vi "AnimatorConfig.vi"(0 "State In":T4 caption="State", 11 "error in (no error)":errorcluster) -> (4 "State Out":T4 caption="State", 8 "Cancel?":bool, 15 "error out":errorcluster)   [LabVIEW 2013, in "AnimatorXControl.xctl"]
uses:
  AnimatorXControl.xctl
  AnimatorState.ctl
  <vilib>/picture/picture.llb/imagedata.ctl
  AnimatorSettings.ctl
  DefaultImageData.vi
  Instance           1 22Saved   AnimatorConfig .vi
panel:
  in  "Cluster":T2
  out "ImageTemp":T3
  out "PathTemp":path
  in  "Reverse":bool
  in  "Frame rate (fps)":dbl
  in  "Animation Settings":enum32{"Automatic", "UseValue"}(radio)
  out "Animation Preview":picture
  in  "Help":bool
  in  "Cancel":bool
  in  "OK":bool
  in  "Down":bool
  in  "Up":bool
  in  "RemoveAll":bool
  in  "Remove":bool
  in  "Add":bool
  in  "Animation Images":i32(listbox)
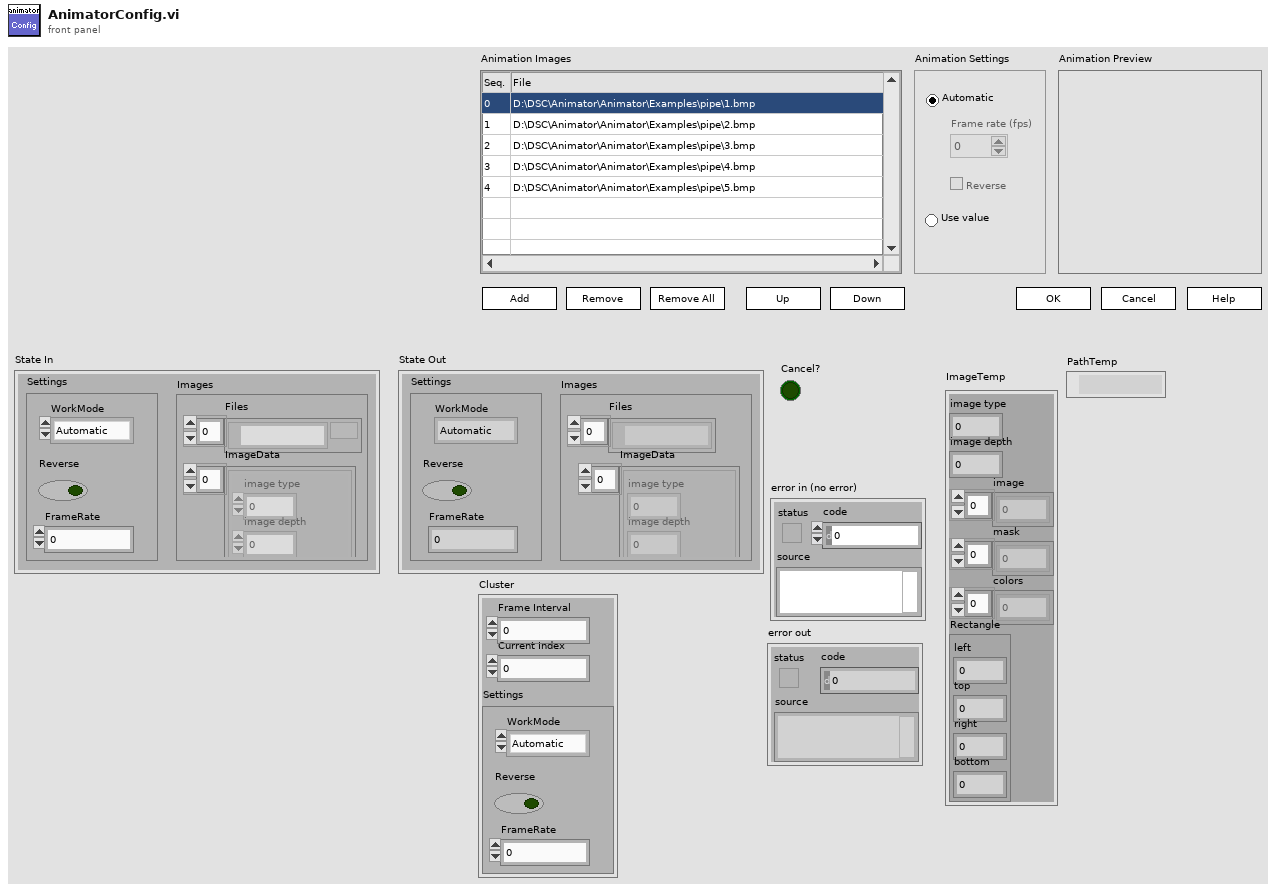
[diagram p1: front panel]
types:
  T1 = typedef "AnimatorXControl.xctl/AnimatorSettings.ctl" = cluster{"Reverse":bool, "FrameRate":dbl, "WorkMode":enum16{"Automatic", "UseValue"}}
  T2 = cluster{"Frame Interval":dbl, "Current Index":u32, "Settings":T1}
  T3 = typedef "imagedata.ctl" = cluster{"image type":i32, "image depth":i32, "image":u8[], "mask":u8[], "colors":u32[], "Rectangle":cluster{"left":i16, "top":i16, "right":i16, "bottom":i16}}
  T4 = typedef "AnimatorXControl.xctl/AnimatorState.ctl" = cluster{"Images":cluster{"Files":path[], "ImageData":T3[]}, "Settings":T1}
  T5 = enum16{"Add", "Remove", "RemoveAll", "MoveUp", "MoveDown"}
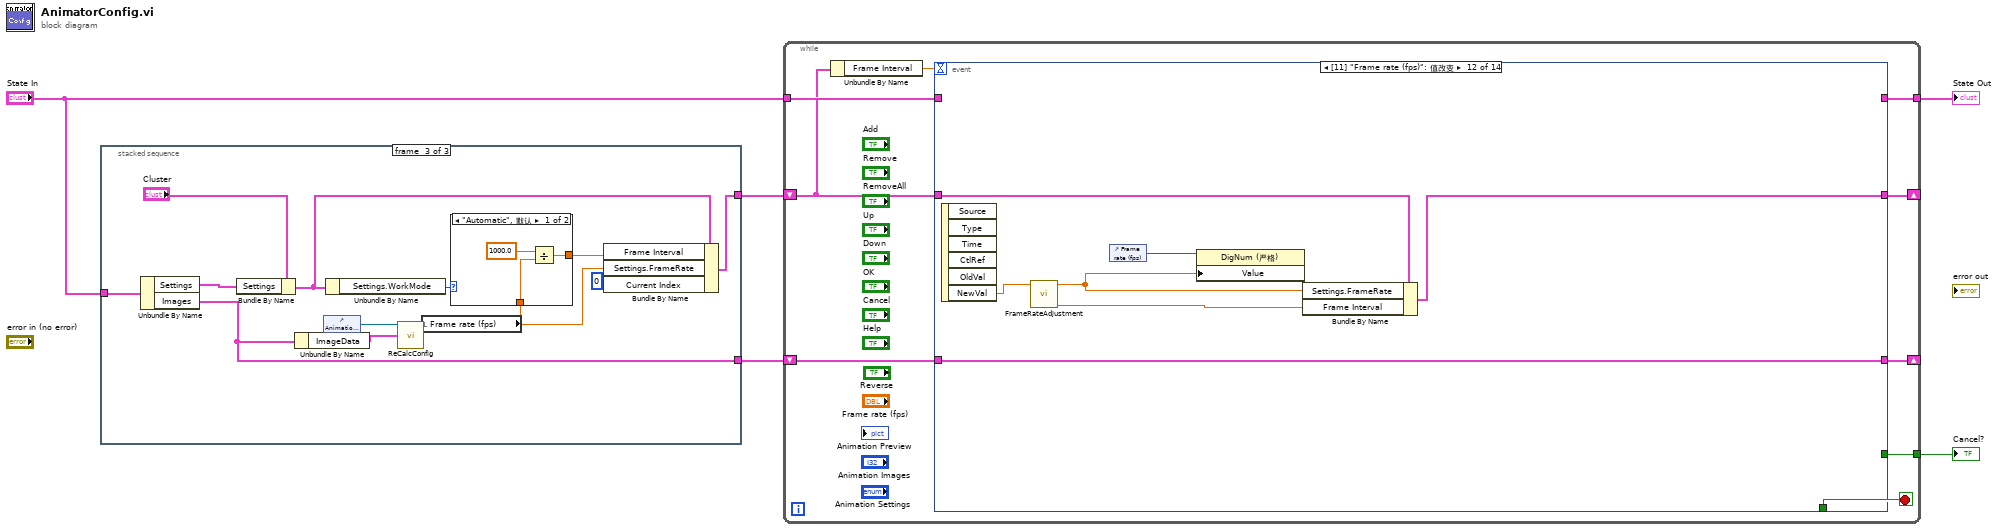
[diagram p0: block diagram]
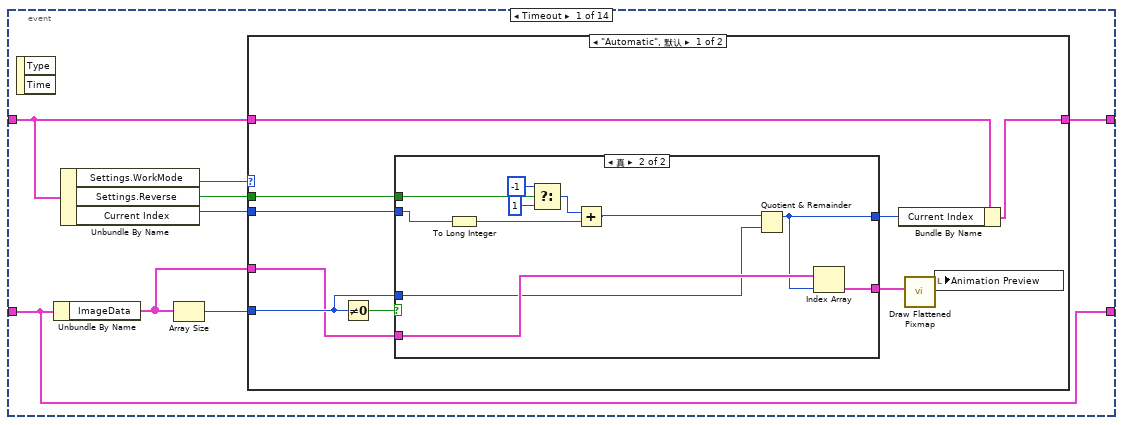
[diagram p2: hidden frame]
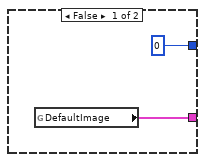
[diagram p3: hidden frame]
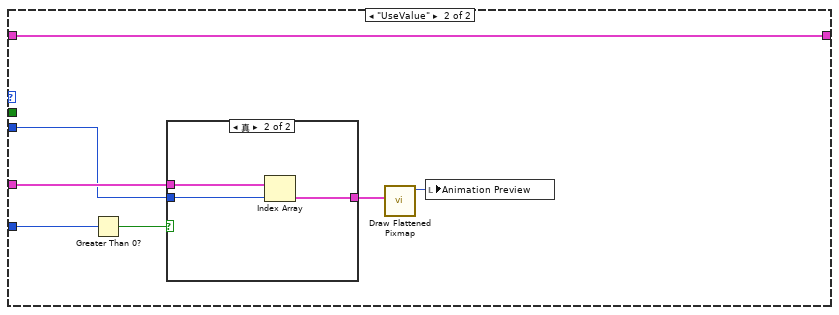
[diagram p4: hidden frame]
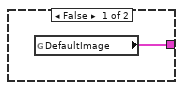
[diagram p5: hidden frame]
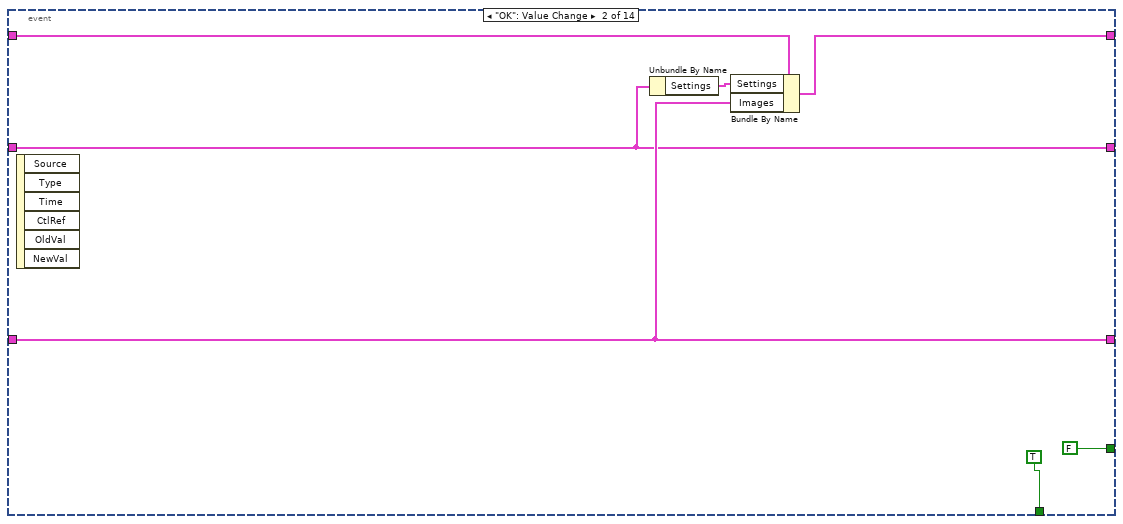
[diagram p6: hidden frame]
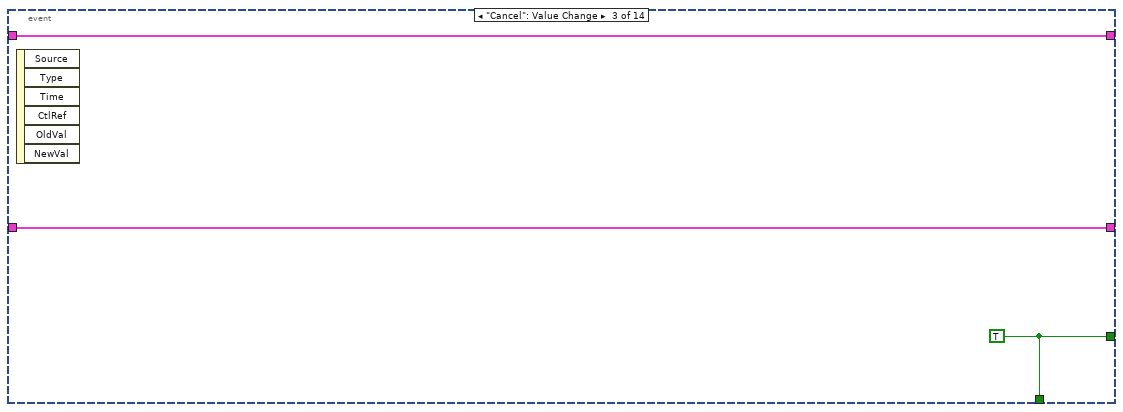
[diagram p7: hidden frame]
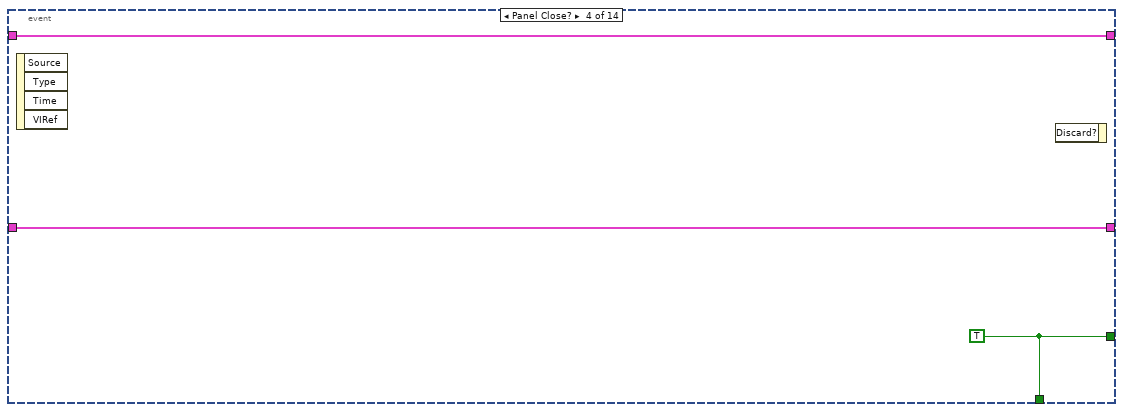
[diagram p8: hidden frame]
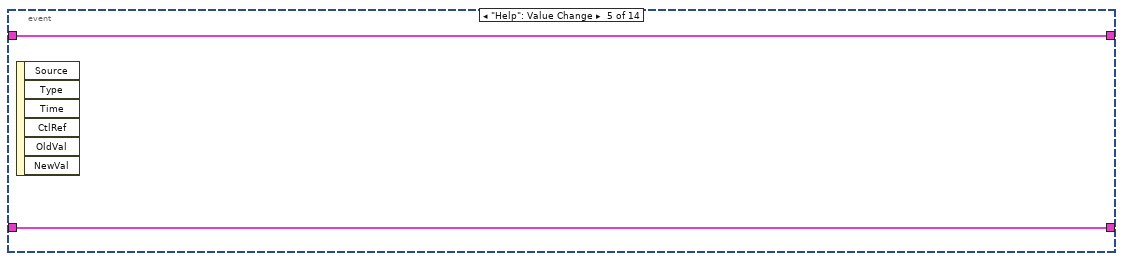
[diagram p9: hidden frame]
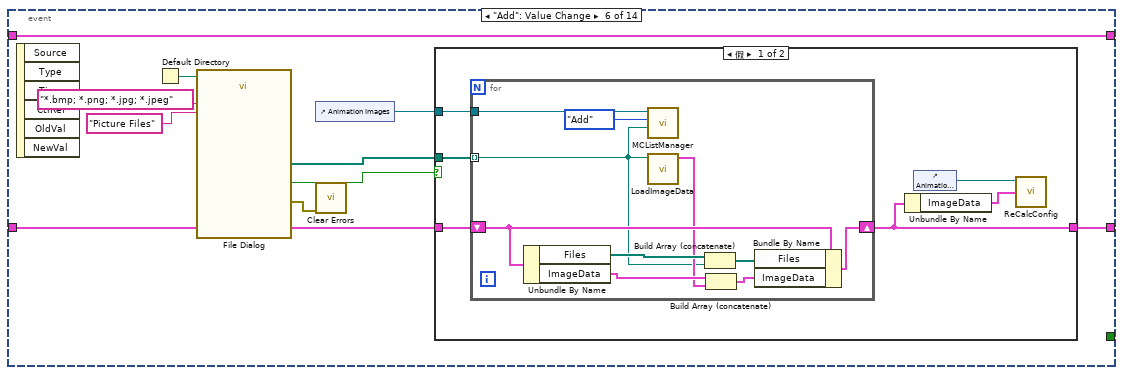
[diagram p10: hidden frame]
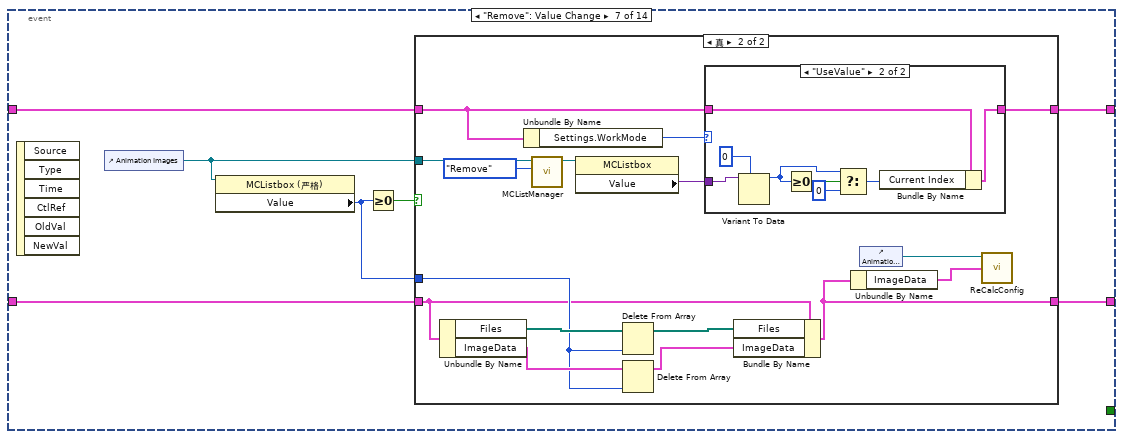
[diagram p12: hidden frame]
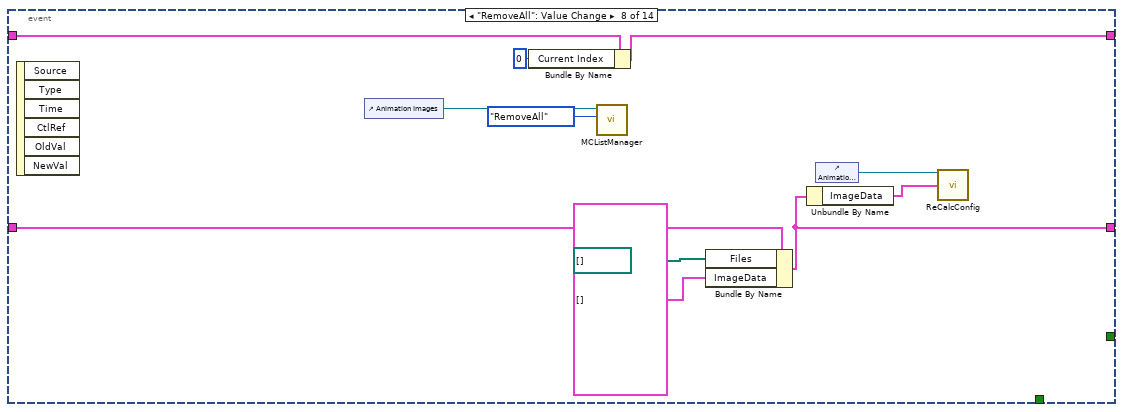
[diagram p15: hidden frame]
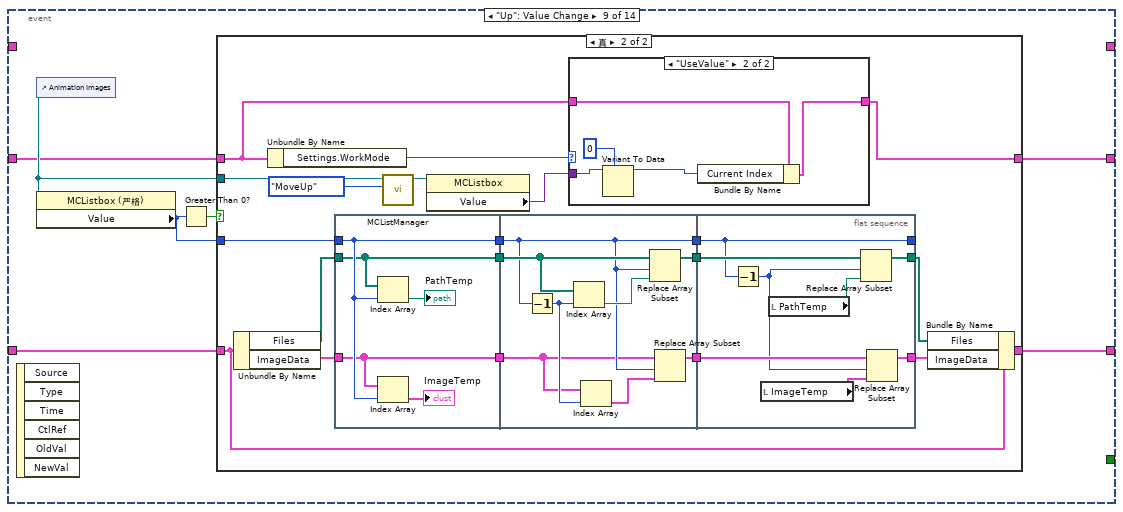
[diagram p16: hidden frame]
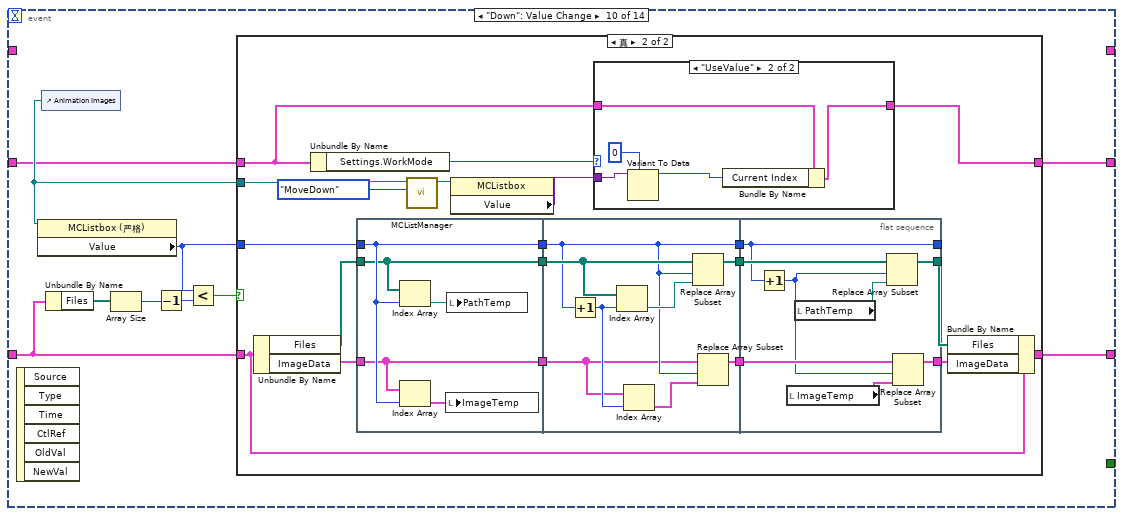
[diagram p19: hidden frame]
diagram:
  n1 = stacked-sequence {
    tunnel: "State In" -> [w22 w31 w46]
    tunnel: [_ _ w44] -> w5
    tunnel: [_ _ w43] -> w4
    frame #0 {
      n2 = Unbundle By Name(w22) -> ("Settings.WorkMode"=w8:enum16{"Automatic", "UseValue"}, "Settings.Reverse"=w17:bool, "Settings.FrameRate"=w11:dbl)
      n3 = case shown="\"UseValue\"" w8 {
        tunnel: [0 ("f") 2 ("t")] -> w7
        tunnel: [enum32{"Automatic", "UseValue"}."Automatic" ("Animation Settings") enum32{"Automatic", "UseValue"}."UseValue" ("Animation Settings")] -> w6
        frame "Automatic", Default {
        }
        frame "UseValue" {
        }
      }
      n4 = local write "Animation Settings"(w6) -> ()
      n5 = control-ref of="Frame rate (fps)"() -> (w21:refnum<vi>)
      n6 = control-ref of="Reverse"() -> (w20:refnum<vi>)
      n7 = Greater?(x=w11, y=25.0) -> (0:w14:bool)
      n8 = Less?(x=w11, y=0.1) -> (x < y?=w13:bool)
      n9 = Not Or(1:w13, 2:w14) -> (0:w10:bool)
      n10 = property class="DigNum (严格)"(reference=w21, "Disabled"=w7) -> (reference out=w19:refnum<vi>)  [unwired: 1 in, 1 out]
      n11 = Select(t=w11, s=w10, f=1.0) -> (s? t:f=w9:dbl)
      n12 = property class="Bool (严格)"(reference=w20, "Disabled"=w7) -> (reference out=w18:refnum<vi>)  [unwired: 1 in, 1 out]
      n13 = property class="DigNum (严格)"(reference=w19, "Value"=w9) -> ()  [unwired: 1 in, 2 out]
      n14 = property class="Bool (严格)"(reference=w18, "Value"=w17) -> ()  [unwired: 1 in, 2 out]
    }
    frame #1 {
      n15 = Unbundle By Name(w31) -> ("Images.Files"=w30:path[])
      n16 = control-ref of="Animation Images"() -> (w29:refnum<vi>)
      n17 = call "MCListManager.vi"("Command"=T5."RemoveAll", "MCListbox Refnum"=w29) -> ("MCListbox Refnum out"=w27:refnum<vi>)  [unwired: 8 in, 1 out]
      n18 = for {
        tunnel: w30 -> [w33] mode=indexing
        tunnel: w27 -> [w34]
        n19 = call "MCListManager.vi"("Path"=w33, "Command"=T5."Add", "MCListbox Refnum"=w34) -> ()  [unwired: 7 in, 2 out]
      }
    }
    frame #2 {
      n20 = Unbundle By Name(w46) -> ("Settings"=w45:T1, "Images"=w43:cluster{"Files":path[], "ImageData":T3[]})
      n21 = Bundle By Name(cluster="Cluster", "Settings"=w45) -> (w42:T2)
      n22 = Unbundle By Name(w43) -> ("ImageData"=w39:T3[])
      n23 = control-ref of="Animation Preview"() -> (w38:refnum<vi>)
      n24 = Unbundle By Name(w42) -> ("Settings.WorkMode"=w37:enum16{"Automatic", "UseValue"})
      n25 = call "ReCalcConfig.vi"("Pict Refnum"=w38, "Image Array"=w39) -> ()  [unwired: 13 in, 1 out]
      n26 = local read "Frame rate (fps)"() -> (w35:dbl)
      n27 = case shown="\"Automatic\", 默认" w37 {
        tunnel: [w49 40.0] -> w36
        tunnel: w35 -> [w48 _]
        frame "Automatic", Default {
          n28 = Divide(x=1000.0, y=w48) -> (x/y=w49:dbl)
        }
        frame "UseValue" {
        }
      }
      n29 = Bundle By Name(cluster=w42, "Frame Interval"=w36, "Settings.FrameRate"=w35, "Current Index"=u32 0) -> (w44:T2)
    }
  }
  n30 = while {
    shift-right: [w57] -> _
    shift-left: w4 -> [w59]
    shift-right: [w58] -> _
    shift-left: w5 -> [w52]
    tunnel: [w55] -> w3
    tunnel: "State In" -> [w54]
    tunnel: [w53] -> w1
    stop <- w56 stop-if-true
    n31 = Unbundle By Name(w52) -> ("Frame Interval"=w51:dbl)
    n32 = event shown="[11] \"Frame rate (fps)\": 值改变" {
      selector: _ -> [_ _ _ _ _ _ _ _ _ _ _ _ _ _]
      dyn-events: _ -> [_ _ _ _ _ _ _ _ _ _ _ _ _ _]
      timeout: w51 -> [_ _ _ _ _ _ _ _ _ _ _ _ _ _]
      tunnel: w52 -> [w64 w103 w111 w114 w116 w124 w145 w184 w190 w246 w307 w334 w339 w342]
      tunnel: w59 -> [w60 w105 w110 w113 w115 w122 w149 w188 w192 w250 w305 w331 w337 w344]
      tunnel: [w63 w103 w111 w114 w116 w124 w144 w182 w189 w245 w306 w333 w338 w341] -> w58
      tunnel: [w60 w105 w110 w113 w115 w121 w148 w185 w191 w251 w305 w331 w337 w344] -> w57
      tunnel: [_ TRUE w109 w112 _ _ _ _ _ _ _ _ _ _] -> w56
      tunnel: [_ FALSE w109 w112 _ _ _ _ _ _ _ _ _ _] -> w55
      tunnel: w54 -> [_ w104 _ _ _ _ _ _ _ _ _ _ _ _]
      tunnel: [_ w106 _ _ _ _ _ _ _ _ _ _ _ _] -> w53
      event Timeout {
        n33 = event-data() -> ()  [unwired: 1 in, 2 out]
        n34 = Unbundle By Name(w60) -> ("ImageData"=w61:T3[])
        n35 = Unbundle By Name(w64) -> ("Settings.WorkMode"=w67:enum16{"Automatic", "UseValue"}, "Settings.Reverse"=w66:bool, "Current Index"=w62:u32)
        n36 = Array Size(array=w61) -> (size(s)=w65:i32)
        n37 = case shown="\"Automatic\", 默认" w67 {
          tunnel: w66 -> [w77 _]
          tunnel: w65 -> [w76 w93]
          tunnel: w61 -> [w75 w92]
          tunnel: w64 -> [w74 w97]
          tunnel: [w73 w97] -> w63
          tunnel: w62 -> [w72 w91]
          frame "Automatic", Default {
            n38 = Not Equal To 0?(x=w76) -> (x != 0?=w71:bool)
            n39 = case shown="真" w71 {
              tunnel: w77 -> [_ w87]
              tunnel: w76 -> [_ w85]
              tunnel: w75 -> [_ w86]
              tunnel: [w79 w84] -> w70
              tunnel: [0 w83] -> w68
              tunnel: w72 -> [_ w82]
              frame False {
                n40 = global read "DefaultImageData.vi" "DefaultImage"() -> (w79:T3)
              }
              frame True {
                n41 = To Long Integer(number=w82) -> (32bit integer=w81:i32)
                n42 = Select(t=-1, s=w87, f=1) -> (s? t:f=w90:i32)
                n43 = Add(x=w90, y=w81) -> (x+y=w80:i32)
                n44 = Quotient & Remainder(x=w80, y=w85) -> (x-y*floor(x/y)=w83:i32)  [unwired: 1 out]
                n45 = Index Array(array=w86, index=w83) -> (element=w84:T3)
              }
            }
            n46 = Bundle By Name(cluster=w74, "Current Index"=w68) -> (w73:T2)
            n47 = call <vilib>:"Draw Flattened Pixmap.vi"("image data"=w70) -> ("new picture"=w69:picture)  [unwired: 8 in]
            n48 = local write "Animation Preview"(w69) -> ()
          }
          frame "UseValue" {
            n49 = Greater Than 0?(x=w93) -> (x > 0?=w94:bool)
            n50 = case shown="真" w94 {
              tunnel: w92 -> [_ w101]
              tunnel: w91 -> [_ w100]
              tunnel: [w98 w99] -> w96
              frame False {
                n51 = global read "DefaultImageData.vi" "DefaultImage"() -> (w98:T3)
              }
              frame True {
                n52 = Index Array(array=w101, index=w100) -> (element=w99:T3)
              }
            }
            n53 = call <vilib>:"Draw Flattened Pixmap.vi"("image data"=w96) -> ("new picture"=w95:picture)  [unwired: 8 in]
            n54 = local write "Animation Preview"(w95) -> ()
          }
        }
      }
      event "OK": Value Change {
        n55 = event-data() -> ()  [unwired: 1 in, 6 out]
        n56 = Unbundle By Name(w103) -> ("Settings"=w107:T1)
        n57 = Bundle By Name(cluster=w104, "Settings"=w107, "Images"=w105) -> (w106:T4)
      }
      event "Cancel": Value Change {
        w109 = TRUE
        n58 = event-data() -> ()  [unwired: 1 in, 6 out]
      }
      event Panel Close? {
        w112 = TRUE
        n59 = event-data() -> ()  [unwired: 1 in, 4 out]
        n60 = event-data() -> ()  [unwired: 2 in, 1 out]
      }
      event "Help": Value Change {
        n61 = event-data() -> ()  [unwired: 1 in, 6 out]
      }
      event "Add": Value Change {
        n62 = event-data() -> ()  [unwired: 1 in, 6 out]
        n63 = Default Directory() -> (w119:path)
        n64 = call "File Dialog"("start path"=w119, "pattern (all files)"="*.bmp; *.png; *.jpg; *.jpeg", "pattern label"="Picture Files") -> ("selected paths"=w123:path[], "cancelled"=w117:bool, "error out"=w118:errorcluster)  [unwired: 9 in, 1 out]
        n65 = control-ref of="Animation Images"() -> (w120:refnum<vi>)
        n66 = call <vilib>:"Clear Errors.vi"("error in (no error)"=w118) -> ()  [unwired: 6 in, 1 out]
        n67 = case shown="假" w117 {
          tunnel: w123 -> [w132 _]
          tunnel: w122 -> [w131 w143]
          tunnel: [w127 w143] -> w121
          tunnel: w120 -> [w130 _]
          frame False {
            n68 = for {
              tunnel: w132 -> [w133] mode=indexing
              shift-right: [w136] -> w127
              shift-left: w131 -> [w140]
              tunnel: w130 -> [w135]
              n69 = Unbundle By Name(w140) -> ("Files"=w141:path[], "ImageData"=w142:T3[])
              n70 = call "MCListManager.vi"("Path"=w133, "Command"=T5."Add", "MCListbox Refnum"=w135) -> ()  [unwired: 7 in, 2 out]
              n71 = call "LoadImageData.vi"("path"=w133) -> ("image data"=w139:T3)  [unwired: 9 in, 1 out]
              n72 = Build Array (concatenate)(w141, w133) -> (w138:path[])
              n73 = Build Array (concatenate)(w142, w139) -> (w137:T3[])
              n74 = Bundle By Name(cluster=w140, "Files"=w138, "ImageData"=w137) -> (w136:cluster{"Files":path[], "ImageData":T3[]})
            }
            n75 = Unbundle By Name(w127) -> ("ImageData"=w129:T3[])
            n76 = control-ref of="Animation Preview"() -> (w128:refnum<vi>)
            n77 = call "ReCalcConfig.vi"("Pict Refnum"=w128, "Image Array"=w129) -> ()  [unwired: 13 in, 1 out]
          }
          frame True {
          }
        }
      }
      event "Remove": Value Change {
        n78 = event-data() -> ()  [unwired: 1 in, 6 out]
        n79 = control-ref of="Animation Images"() -> (w147:refnum<vi>)
        n80 = property class="MCListbox (严格)"(reference=w147) -> ("Value"=w146:i32)  [unwired: 1 in, 2 out]
        n81 = Greater Or Equal To 0?(x=w146) -> (x >= 0?=w150:bool)
        n82 = case shown="真" w150 {
          tunnel: w149 -> [w152 w163]
          tunnel: [w152 w160] -> w148
          tunnel: w147 -> [_ w167]
          tunnel: w146 -> [_ w164]
          tunnel: w145 -> [w151 w157]
          tunnel: [w151 w156] -> w144
          frame False {
          }
          frame True {
            n83 = Unbundle By Name(w163) -> ("Files"=w166:path[], "ImageData"=w165:T3[])
            n84 = Unbundle By Name(w157) -> ("Settings.WorkMode"=w158:enum16{"Automatic", "UseValue"})
            n85 = call "MCListManager.vi"("Command"=T5."Remove", "MCListbox Refnum"=w167) -> ("MCListbox Refnum out"=w159:refnum<vi>)  [unwired: 8 in, 1 out]
            n86 = property class="MCListbox"(reference=w159) -> ("Value"=w155:variant)  [unwired: 1 in, 2 out]
            n87 = Delete From Array(array=w166, index=w164) -> (array with subset deleted=w162:path[])  [unwired: 1 in, 1 out]
            n88 = Delete From Array(array=w165, index=w164) -> (array with subset deleted=w161:T3[])  [unwired: 1 in, 1 out]
            n89 = case shown="\"UseValue\"" w158 {
              tunnel: w157 -> [w169 w175]
              tunnel: [w169 w174] -> w156
              tunnel: w155 -> [_ w177]
              frame "Automatic", Default {
              }
              frame "UseValue" {
                n90 = Variant To Data(type=0, Variant=w177) -> (data=w171:i32)  [unwired: 1 in, 1 out]
                n91 = Greater Or Equal To 0?(x=w171) -> (x >= 0?=w173:bool)
                n92 = Select(t=w171, s=w173, f=0) -> (s? t:f=w172:i32)
                n93 = Bundle By Name(cluster=w175, "Current Index"=w172) -> (w174:T2)
              }
            }
            n94 = Bundle By Name(cluster=w163, "Files"=w162, "ImageData"=w161) -> (w160:cluster{"Files":path[], "ImageData":T3[]})
            n95 = Unbundle By Name(w160) -> ("ImageData"=w153:T3[])
            n96 = control-ref of="Animation Preview"() -> (w154:refnum<vi>)
            n97 = call "ReCalcConfig.vi"("Pict Refnum"=w154, "Image Array"=w153) -> ()  [unwired: 13 in, 1 out]
          }
        }
      }
      event "RemoveAll": Value Change {
        n98 = event-data() -> ()  [unwired: 1 in, 6 out]
        n99 = control-ref of="Animation Images"() -> (w187:refnum<vi>)
        n100 = Bundle By Name(cluster=w184, "Current Index"=u32 0) -> (w182:T2)
        n101 = call "MCListManager.vi"("Command"=T5."RemoveAll", "MCListbox Refnum"=w187) -> ()  [unwired: 8 in, 2 out]
        n102 = Bundle By Name(cluster=w188, "Files"=path[] [], "ImageData"=T3[] []) -> (w185:cluster{"Files":path[], "ImageData":T3[]})
        n103 = Unbundle By Name(w185) -> ("ImageData"=w178:T3[])
        n104 = control-ref of="Animation Preview"() -> (w179:refnum<vi>)
        n105 = call "ReCalcConfig.vi"("Pict Refnum"=w179, "Image Array"=w178) -> ()  [unwired: 13 in, 1 out]
      }
      event "Up": Value Change {
        n106 = event-data() -> ()  [unwired: 1 in, 6 out]
        n107 = control-ref of="Animation Images"() -> (w194:refnum<vi>)
        n108 = property class="MCListbox (严格)"(reference=w194) -> ("Value"=w193:i32)  [unwired: 1 in, 2 out]
        n109 = Greater Than 0?(x=w193) -> (x > 0?=w195:bool)
        n110 = case shown="真" w195 {
          tunnel: w194 -> [_ w216]
          tunnel: w193 -> [_ w214]
          tunnel: w192 -> [w197 w203]
          tunnel: [w197 w204] -> w191
          tunnel: w190 -> [w196 w199]
          tunnel: [w196 w198] -> w189
          frame False {
          }
          frame True {
            n111 = Unbundle By Name(w203) -> ("Files"=w208:path[], "ImageData"=w207:T3[])
            n112 = Unbundle By Name(w199) -> ("Settings.WorkMode"=w202:enum16{"Automatic", "UseValue"})
            n113 = flat-sequence {
              tunnel: [w228] -> w215
              tunnel: w214 -> [w228]
              tunnel: w208 -> [w225]
              tunnel: w207 -> [w224]
              tunnel: [w225] -> w212
              tunnel: [w224] -> w211
              tunnel: w215 -> [w233]
              tunnel: [w233] -> w213
              tunnel: w212 -> [w235]
              tunnel: w211 -> [w231]
              tunnel: [w230] -> w210
              tunnel: [w229] -> w209
              tunnel: [w242] -> _
              tunnel: w213 -> [w242]
              tunnel: w210 -> [w244]
              tunnel: w209 -> [w243]
              tunnel: [w238] -> w205
              tunnel: [w237] -> w206
              frame #0 {
                n114 = Index Array(array=w225, index=w228) -> (element=→"PathTemp":path)
                n115 = Index Array(array=w224, index=w228) -> (element=→"ImageTemp":T3)
              }
              frame #1 {
                n116 = Decrement(x=w233) -> (x-1=w236:i32)
                n117 = Index Array(array=w235, index=w236) -> (element=w234:path)
                n118 = Index Array(array=w231, index=w236) -> (element=w232:T3)
                n119 = Replace Array Subset(array=w235, new element=w234, index=w233) -> (w230:path[])
                n120 = Replace Array Subset(array=w231, new element=w232, index=w233) -> (w229:T3[])
              }
              frame #2 {
                n121 = Decrement(x=w242) -> (x-1=w241:i32)
                n122 = local read "ImageTemp"() -> (w239:T3)
                n123 = local read "PathTemp"() -> (w240:path)
                n124 = Replace Array Subset(array=w244, new element=w240, index=w241) -> (w238:path[])
                n125 = Replace Array Subset(array=w243, new element=w239, index=w241) -> (w237:T3[])
              }
            }
            n126 = call "MCListManager.vi"("Command"=T5."MoveUp", "MCListbox Refnum"=w216) -> ("MCListbox Refnum out"=w201:refnum<vi>)  [unwired: 8 in, 1 out]
            n127 = property class="MCListbox"(reference=w201) -> ("Value"=w200:variant)  [unwired: 1 in, 2 out]
            n128 = case shown="\"UseValue\"" w202 {
              tunnel: w199 -> [w218 w221]
              tunnel: [w218 w219] -> w198
              tunnel: w200 -> [_ w223]
              frame "Automatic", Default {
              }
              frame "UseValue" {
                n129 = Variant To Data(type=0, Variant=w223) -> (data=w220:i32)  [unwired: 1 in, 1 out]
                n130 = Bundle By Name(cluster=w221, "Current Index"=w220) -> (w219:T2)
              }
            }
            n131 = Bundle By Name(cluster=w203, "Files"=w205, "ImageData"=w206) -> (w204:cluster{"Files":path[], "ImageData":T3[]})
          }
        }
      }
      event "Down": Value Change {
        n132 = event-data() -> ()  [unwired: 1 in, 6 out]
        n133 = control-ref of="Animation Images"() -> (w247:refnum<vi>)
        n134 = property class="MCListbox (严格)"(reference=w247) -> ("Value"=w249:i32)  [unwired: 1 in, 2 out]
        n135 = Unbundle By Name(w250) -> ("Files"=w254:path[])
        n136 = Array Size(array=w254) -> (size(s)=w253:i32)
        n137 = Decrement(x=w253) -> (x-1=w252:i32)
        n138 = Less?(x=w249, y=w252) -> (x < y?=w248:bool)
        n139 = case shown="真" w248 {
          tunnel: w247 -> [_ w275]
          tunnel: w249 -> [_ w273]
          tunnel: w250 -> [w256 w262]
          tunnel: [w256 w263] -> w251
          tunnel: w246 -> [w255 w260]
          tunnel: [w255 w257] -> w245
          frame False {
          }
          frame True {
            n140 = Unbundle By Name(w262) -> ("Files"=w267:path[], "ImageData"=w266:T3[])
            n141 = Unbundle By Name(w260) -> ("Settings.WorkMode"=w259:enum16{"Automatic", "UseValue"})
            n142 = flat-sequence {
              tunnel: [w287] -> w274
              tunnel: w273 -> [w287]
              tunnel: w267 -> [w286]
              tunnel: w266 -> [w285]
              tunnel: [w286] -> w271
              tunnel: [w285] -> w270
              tunnel: w274 -> [w292]
              tunnel: [w292] -> w272
              tunnel: w271 -> [w294]
              tunnel: w270 -> [w290]
              tunnel: [w289] -> w269
              tunnel: [w288] -> w268
              tunnel: [w301] -> _
              tunnel: w272 -> [w301]
              tunnel: w269 -> [w303]
              tunnel: w268 -> [w302]
              tunnel: [w297] -> w264
              tunnel: [w296] -> w265
              frame #0 {
                n143 = Index Array(array=w286, index=w287) -> (element=w284:path)
                n144 = Index Array(array=w285, index=w287) -> (element=w283:T3)
                n145 = local write "ImageTemp"(w283) -> ()
                n146 = local write "PathTemp"(w284) -> ()
              }
              frame #1 {
                n147 = Increment(x=w292) -> (x+1=w295:i32)
                n148 = Index Array(array=w294, index=w295) -> (element=w293:path)
                n149 = Index Array(array=w290, index=w295) -> (element=w291:T3)
                n150 = Replace Array Subset(array=w294, new element=w293, index=w292) -> (w289:path[])
                n151 = Replace Array Subset(array=w290, new element=w291, index=w292) -> (w288:T3[])
              }
              frame #2 {
                n152 = Increment(x=w301) -> (x+1=w300:i32)
                n153 = local read "ImageTemp"() -> (w298:T3)
                n154 = local read "PathTemp"() -> (w299:path)
                n155 = Replace Array Subset(array=w303, new element=w299, index=w300) -> (w297:path[])
                n156 = Replace Array Subset(array=w302, new element=w298, index=w300) -> (w296:T3[])
              }
            }
            n157 = call "MCListManager.vi"("Command"=T5."MoveDown", "MCListbox Refnum"=w275) -> ("MCListbox Refnum out"=w261:refnum<vi>)  [unwired: 8 in, 1 out]
            n158 = property class="MCListbox"(reference=w261) -> ("Value"=w258:variant)  [unwired: 1 in, 2 out]
            n159 = case shown="\"UseValue\"" w259 {
              tunnel: w260 -> [w277 w280]
              tunnel: [w277 w278] -> w257
              tunnel: w258 -> [_ w282]
              frame "Automatic", Default {
              }
              frame "UseValue" {
                n160 = Variant To Data(type=0, Variant=w282) -> (data=w279:i32)  [unwired: 1 in, 1 out]
                n161 = Bundle By Name(cluster=w280, "Current Index"=w279) -> (w278:T2)
              }
            }
            n162 = Bundle By Name(cluster=w262, "Files"=w264, "ImageData"=w265) -> (w263:cluster{"Files":path[], "ImageData":T3[]})
          }
        }
      }
      event "Animation Settings": Value Change {
        n163 = event-data() -> ("NewVal"=w310:enum32{"Automatic", "UseValue"})  [unwired: 1 in, 5 out]
        n164 = case shown="\"UseValue\"" w310 {
          tunnel: [0 ("f") 2 ("f")] -> w304
          tunnel: w307 -> [w317 w327]
          tunnel: [w316 w326] -> w306
          frame "Automatic", Default {
            n165 = local read "Frame rate (fps)"() -> (w314:dbl)
            n166 = Divide(x=1000.0, y=w314) -> (x/y=w313:dbl)
            n167 = Bundle By Name(cluster=w317, "Frame Interval"=w313, "Settings.FrameRate"=w314, "Settings.WorkMode"=enum16{"Automatic", "UseValue"}."Automatic") -> (w316:T2)
          }
          frame "UseValue" {
            n168 = control-ref of="Animation Images"() -> (w321:refnum<vi>)
            n169 = property class="MCListbox (严格)"(reference=w321) -> ("Value"=w324:i32)  [unwired: 1 in, 2 out]
            n170 = Greater Or Equal To 0?(x=w324) -> (x >= 0?=w325:bool)
            n171 = Select(t=w324, s=w325, f=0) -> (s? t:f=w322:i32)
            n172 = Bundle By Name(cluster=w327, "Frame Interval"=40.0, "Current Index"=w322, "Settings.WorkMode"=enum16{"Automatic", "UseValue"}."UseValue") -> (w326:T2)
          }
        }
        n173 = control-ref of="Frame rate (fps)"() -> (w309:refnum<vi>)
        n174 = control-ref of="Reverse"() -> (w308:refnum<vi>)
        n175 = property class="DigNum (严格)"(reference=w309, "Disabled"=w304) -> ()  [unwired: 1 in, 2 out]
        n176 = property class="Bool (严格)"(reference=w308, "Disabled"=w304) -> ()  [unwired: 1 in, 2 out]
      }
      event "Frame rate (fps)": Value Change {
        n177 = event-data() -> ("NewVal"=w330:dbl)  [unwired: 1 in, 5 out]
        n178 = call "FrameRateAdjustment.vi"("FrameRate In"=w330) -> ("FrameInterval"=w328:dbl, "FrameRate Out"=w329:dbl)  [unwired: 9 in]
        n179 = control-ref of="Frame rate (fps)"() -> (w332:refnum<vi>)
        n180 = property class="DigNum (严格)"(reference=w332, "Value"=w329) -> ()  [unwired: 1 in, 2 out]
        n181 = Bundle By Name(cluster=w334, "Settings.FrameRate"=w329, "Frame Interval"=w328) -> (w333:T2)
      }
      event "Reverse": Value Change {
        n182 = event-data() -> ("NewVal"=w335:bool)  [unwired: 1 in, 5 out]
        n183 = Bundle By Name(cluster=w339, "Settings.Reverse"=w335) -> (w338:T2)
        n184 = control-ref of="Reverse"() -> (w336:refnum<vi>)
        n185 = property class="Bool (严格)"(reference=w336, "Value"=w335) -> ()  [unwired: 1 in, 2 out]
      }
      event "Animation Images": Value Change {
        n186 = event-data() -> ("NewVal"=w340:i32)  [unwired: 1 in, 5 out]
        n187 = Unbundle By Name(w342) -> ("Settings.WorkMode"=w343:enum16{"Automatic", "UseValue"})
        n188 = case shown="\"UseValue\"" w343 {
          tunnel: w342 -> [w345 w348]
          tunnel: [w345 w351] -> w341
          tunnel: w340 -> [_ w346]
          frame "Automatic", Default {
          }
          frame "UseValue" {
            n189 = Unbundle By Name(w348) -> ("Current Index"=w347:u32)
            n190 = Less Than 0?(x=w346) -> (x < 0?=w349:bool)
            n191 = Select(t=w347, s=w349, f=w346) -> (s? t:f=w350:u32)
            n192 = Bundle By Name(cluster=w348, "Current Index"=w350) -> (w351:T2)
          }
        }
      }
    }
  }
  "State Out" <- w1
  "Cancel?" <- w3
